vi "Get Label Data.vi"(10 "expmode":i32, 11 "scanmode":i32) -> (2 "found?":bool, 3 "data":T1)   [LabVIEW 2009]
uses:
  Global/Set Up.vi
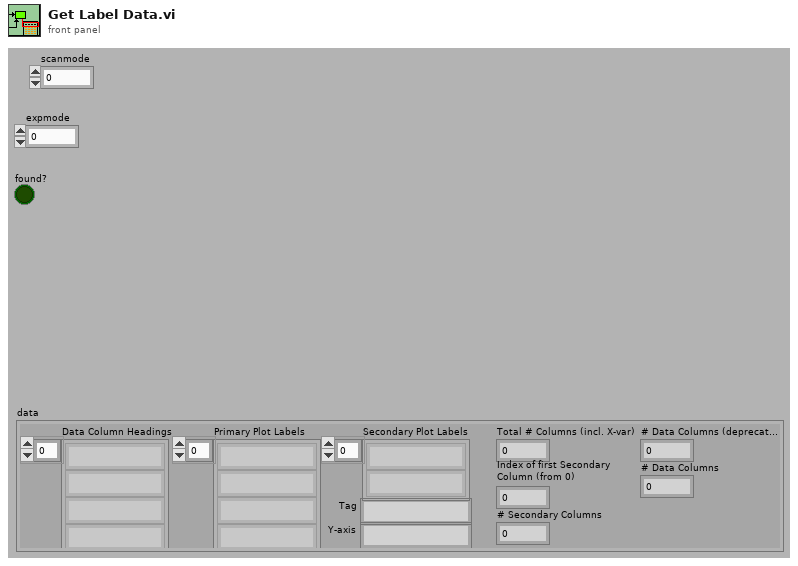
[diagram p1: front panel]
types:
  T1 = cluster{"Data Column Headings":string[], "Primary Plot Labels":string[], "Secondary Plot Labels":string[], "Tag":string, "Y-axis":string, "Total # Columns (incl. X-var)":dbl, "Index of first Secondary\nColumn (from 0)":dbl, "# Secondary Columns":dbl, "# Data Columns (deprecated)":dbl, "# Data Columns":dbl}
  T2 = cluster{"Data Column Headings":string[], "Primary Plot Labels":string[], "Secondary Plot Labels":string[], "Tag":string, "Y-axis":string, "Total # Columns (incl. X-var)":dbl, "Index of first Secondary\nColumn (from 0)":dbl, "# Secondary Columns":dbl, "# Data Columns (deprecated)":dbl, "# Data Columns":dbl}[]
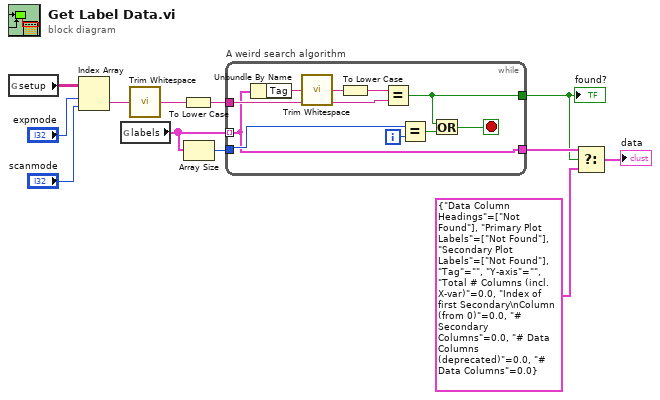
[diagram p0: block diagram]
diagram:
  n1 = global read "Set Up.vi" "setup"() -> (w10:string[][])
  n2 = Index Array(array=w10, index (row)="expmode", index (col)="scanmode") -> (element=w3:string)
  n3 = global read "Set Up.vi" "labels"() -> (w4:T2)
  n4 = call <vilib>:"Trim Whitespace.vi"("string"=w3) -> ("trimmed string"=w5:string)  [unwired: 1 in]
  n5 = To Lower Case(string=w5) -> (all lower case string=w6:string)
  n6 = Array Size(array=w4) -> (size(s)=w7:i32)
  n7 = while "A weird search algorithm" {
    tunnel: w4 -> [w13] mode=indexing
    tunnel: w6 -> [w19]
    tunnel: w7 -> [w18]
    tunnel: [w14] -> w2
    tunnel: [w13] -> w8
    i -> [w17]
    stop <- w15 stop-if-true
    n8 = Unbundle By Name(w13) -> ("Tag"=w21:string)
    n9 = call <vilib>:"Trim Whitespace.vi"("string"=w21) -> ("trimmed string"=w22:string)  [unwired: 1 in]
    n10 = To Lower Case(string=w22) -> (all lower case string=w20:string)
    n11 = Equal?(x=w20, y=w19) -> (x = y?=w14:bool)
    n12 = Equal?(x=w18, y=w17) -> (x = y?=w16:bool)
    n13 = Or(x=w14, y=w16) -> (x .or. y?=w15:bool)
  }
  "found?" <- w2
  n14 = Select(t=w8, s=w2, f=T1 {"Data Column Headings"=["Not Found"], "Primary Plot Labels"=["Not Found"], "Secondary Plot Labels"=["Not Found"], "Tag"="", "Y-axis"="", "Total # Columns (incl. X-var)"=0.0, "Index of first Secondary\nColumn (from 0)"=0.0, "# Secondary Columns"=0.0, "# Data Columns (deprecated)"=0.0, "# Data Columns"=0.0} ("data 2")) -> (s? t:f=→"data":T1)
